vi "initial angle.vi"() -> ()   [LabVIEW 2019]
panel:
  in  "Boolean":bool
  in  "Numeric":dbl
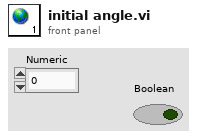
[diagram p1: front panel]
diagram:
